vi "Distance Drive PID.vi"(4 "reinitialize? (F)":bool, 5 "output range":cluster{"output high":dbl, "output low":dbl}={"output high"=100.0, "output low"=-100.0} {"output low" format="%.2f"; "output high" format="%.2f"}, 6 "PID Params":T1, 7 "Setpoint":dbl, 8 "Max Stop Speed":dbl, 9 "Distance Stop":dbl, 10 "Current Speed":dbl, 11 "Current Distance":dbl) -> (0 "Finished":bool, 2 "output":dbl)   [LabVIEW 2015]
uses:
  <vilib>/addons/control/pid/pid.llb/PID (DBL).vi
  <vilib>/addons/control/pid/NI_PID_pid.lvlib
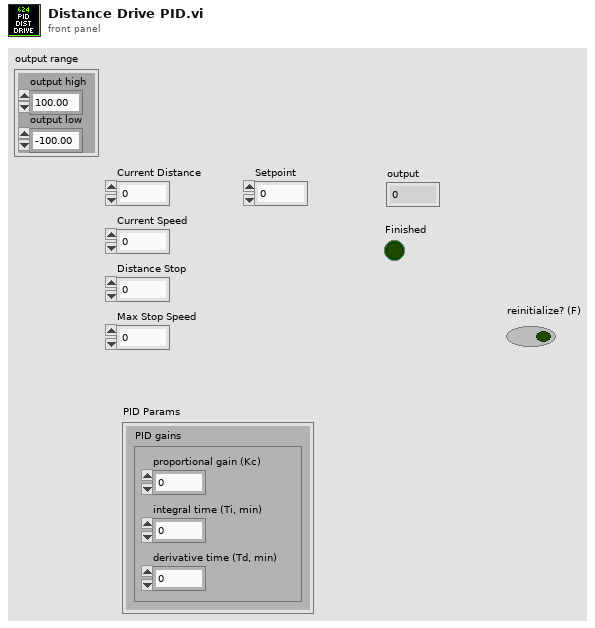
[diagram p1: front panel]
types:
  T1 = cluster{"PID gains":cluster{"proportional gain (Kc)":dbl, "integral time (Ti, min)":dbl, "derivative time (Td, min)":dbl}}
  T2 = cluster{"proportional gain (Kc)":dbl, "integral time (Ti, min)":dbl, "derivative time (Td, min)":dbl}
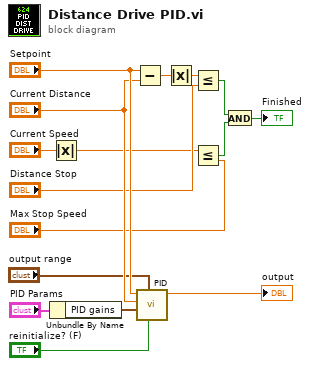
[diagram p0: block diagram]
diagram:
  n1 = Unbundle By Name("PID Params") -> ("PID gains"=w15:T2)
  n2 = Absolute Value(x="Current Speed") -> (abs(x)=w5:dbl)
  n3 = Subtract(x="Setpoint", y="Current Distance") -> (x-y=w10:dbl)
  n4 = call-poly <vilib>:"PID.vi"("reinitialize? (F)"="reinitialize? (F)", "output range"="output range", "PID gains"=w15, "process variable"="Current Distance", "setpoint"="Setpoint") -> ("output"=→"output":dbl)  [unwired: 5 in, 1 out]
  n5 = Absolute Value(x=w10) -> (abs(x)=w8:dbl)
  n6 = Less Or Equal?(x=w8, y="Distance Stop") -> (x <= y?=w4:bool)
  n7 = Less Or Equal?(x=w5, y="Max Stop Speed") -> (x <= y?=w3:bool)
  n8 = And(x=w4, y=w3) -> (x .and. y?=→"Finished":bool)
